vi "TemperatureDAQExample.vi"() -> ()   [LabVIEW 2024]
uses:
  <vilib>/Analysis/baseanly.llb/Mean (DBL).vi
  <vilib>/DAQmx/create/channels.llb/DAQmx Create Channel (AI-Temperature-Thermocouple).vi
  <vilib>/DAQmx/configure/trigger.llb/DAQmx Start Trigger (Digital Edge).vi
  <vilib>/Analysis/NI_AALBase.lvlib
  <vilib>/Utility/TDMS File Viewer/NI_TDMS File Viewer.lvlib
panel:
  out "data 4":dynamicdata(graph) caption="data"
  out "data 3":dynamicdata(graph) caption="data"
  out "mean":dbl format="%0.2f"
  in  "Boolean":bool
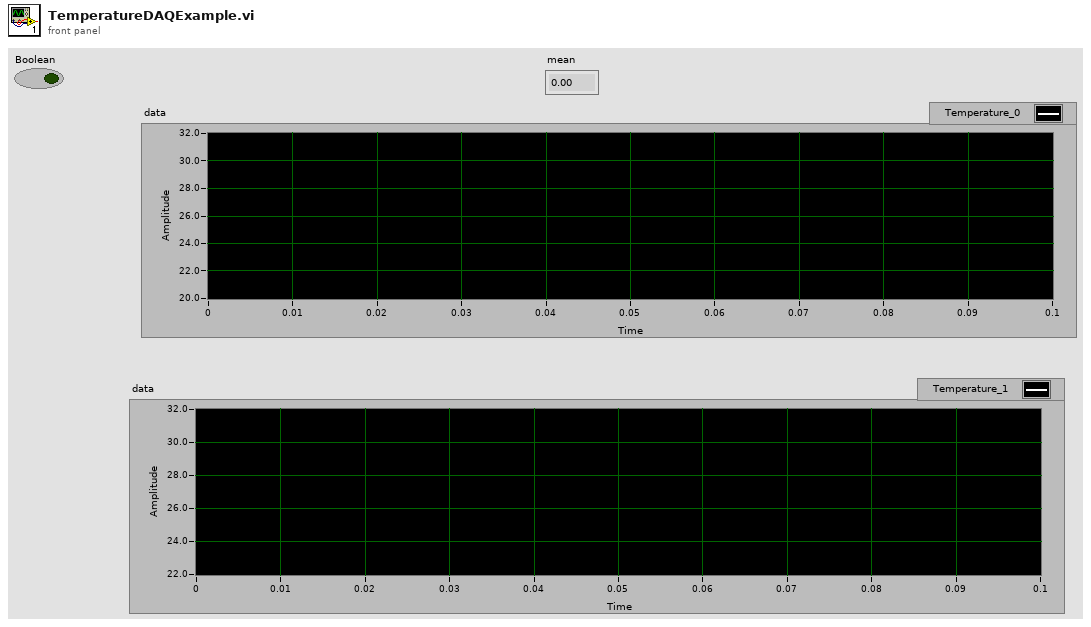
[diagram p1: front panel]
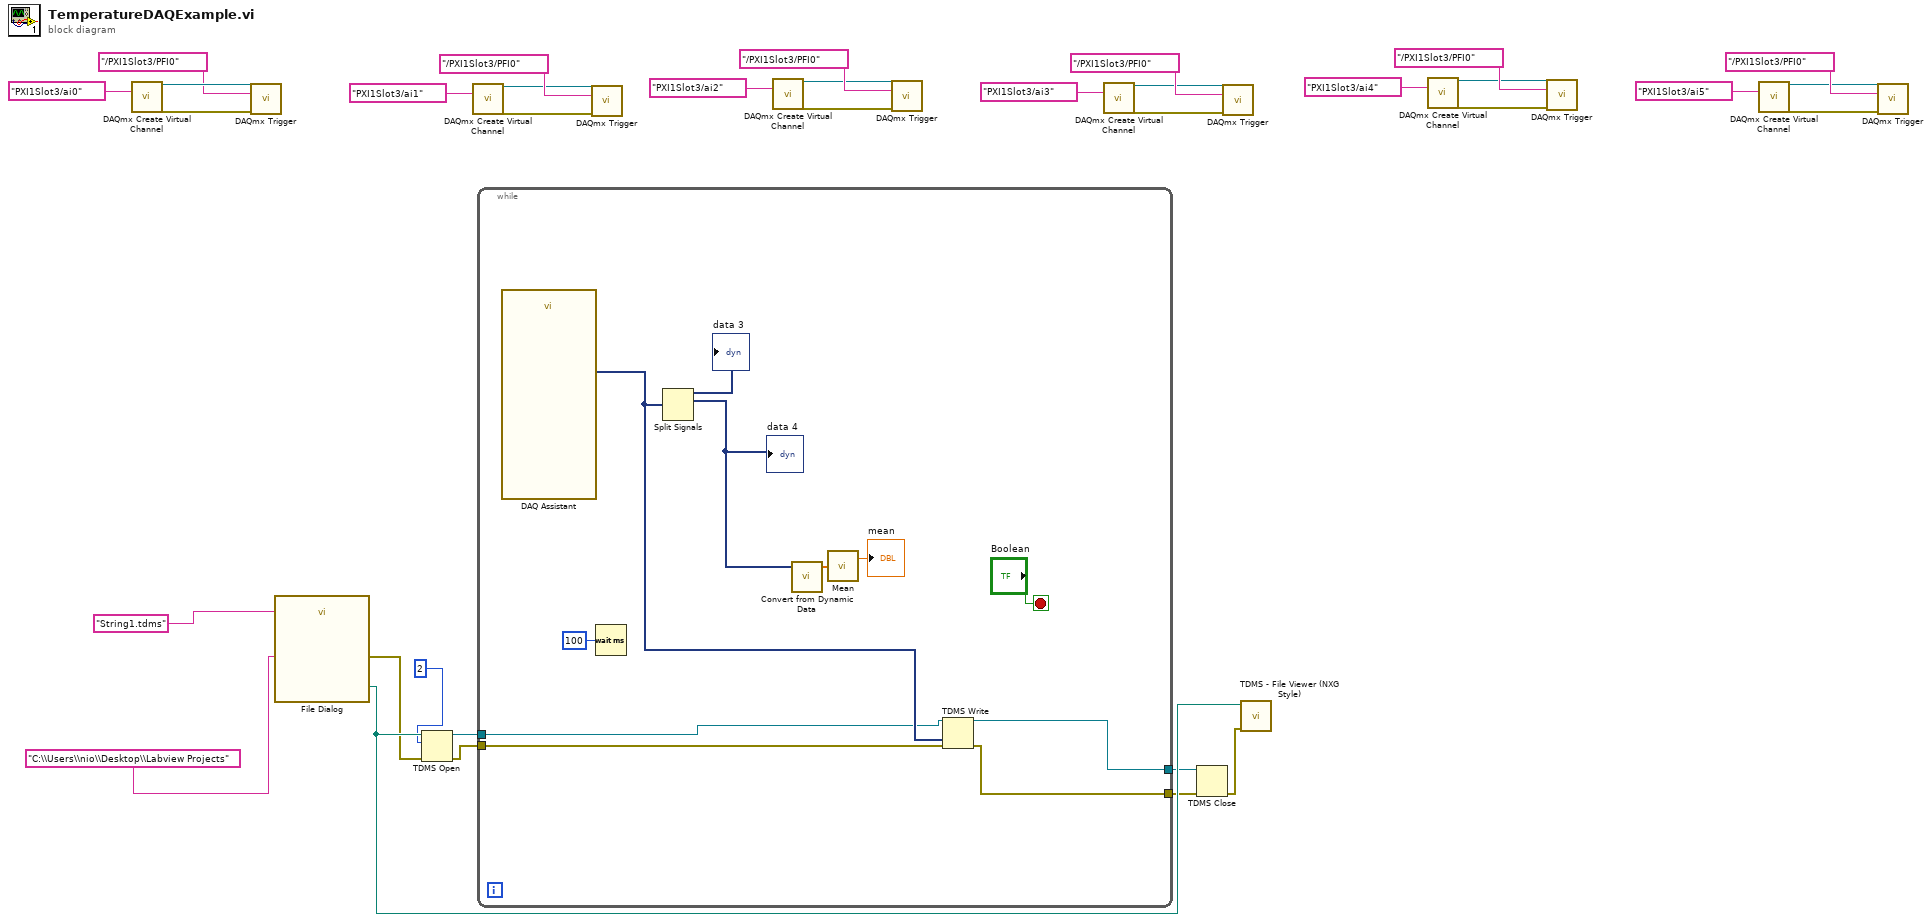
[diagram p0: block diagram]
diagram:
  n1 = call-poly <vilib>:"DAQmx Create Virtual Channel.vi"("physical channels"=tag "PXI1Slot3/ai0") -> ("task out"=w33:refnum<k21>, "error out"=w32:errorcluster)  [unwired: 13 in]
  n2 = call-poly <vilib>:"DAQmx Trigger.vi"("task/channels in"=w33, "source"=tag "/PXI1Slot3/PFI0", "error in"=w32) -> ()  [unwired: 11 in, 2 out]
  n3 = call "File Dialog"("prompt"="C:\\Users\\nio\\Desktop\\Labview Projects", "default name"="String1.tdms") -> ("selected path"=w24:path, "error out"=w23:errorcluster)  [unwired: 10 in, 2 out]
  n4 = TDMS Open(8:w23, 10:u32 2 ("milliseconds to wait"), 11:w24) -> (0:w21:errorcluster, 3:w20:refnum<k34>)  [unwired: 4 in]
  n5 = call-poly <vilib>:"DAQmx Create Virtual Channel.vi"("physical channels"=tag "PXI1Slot3/ai1") -> ("task out"=w27:refnum<k21>, "error out"=w29:errorcluster)  [unwired: 13 in]
  n6 = while {
    tunnel: w21 -> [w38]
    tunnel: w20 -> [w37]
    tunnel: [w36] -> w19
    tunnel: [w35] -> w18
    stop <- "Boolean" stop-if-true
    n7 = call "DAQ Assistant"() -> ("data"=w39:dynamicdata)  [unwired: 17 in, 2 out]
    n8 = Wait (ms)(milliseconds to wait=u32 100) -> ()  [unwired: 1 out]
    n9 = Split Signals(w39) -> (→"data 3":dynamicdata, w40:dynamicdata)  [unwired: 4 in, 2 out]
    "data 4" <- w40
    n10 = call "Convert from Dynamic Data"("Dynamic Data Type"=w40) -> ("Array"=w43:dbl[])  [unwired: 3 in]
    n11 = call-poly <vilib>:"Mean.vi"("X"=w43) -> ("mean"=→"mean":dbl)  [unwired: 1 out]
    n12 = TDMS Write(0:w37, 9:w39, 11:w38) -> (4:w35:refnum<k34>, 15:w36:errorcluster)  [unwired: 3 in, 2 out]
  }
  n13 = call-poly <vilib>:"DAQmx Trigger.vi"("task/channels in"=w27, "source"=tag "/PXI1Slot3/PFI0", "error in"=w29) -> ()  [unwired: 11 in, 2 out]
  n14 = call-poly <vilib>:"DAQmx Create Virtual Channel.vi"("physical channels"=tag "PXI1Slot3/ai2") -> ("task out"=w13:refnum<k21>, "error out"=w15:errorcluster)  [unwired: 13 in]
  n15 = call-poly <vilib>:"DAQmx Trigger.vi"("task/channels in"=w13, "source"=tag "/PXI1Slot3/PFI0", "error in"=w15) -> ()  [unwired: 11 in, 2 out]
  n16 = call-poly <vilib>:"DAQmx Create Virtual Channel.vi"("physical channels"=tag "PXI1Slot3/ai3") -> ("task out"=w9:refnum<k21>, "error out"=w11:errorcluster)  [unwired: 13 in]
  n17 = TDMS Close(8:w19, 11:w18) -> (0:w17:errorcluster)  [unwired: 1 out]
  n18 = call-poly <vilib>:"DAQmx Trigger.vi"("task/channels in"=w9, "source"=tag "/PXI1Slot3/PFI0", "error in"=w11) -> ()  [unwired: 11 in, 2 out]
  n19 = call <vilib>:"TDMS - File Viewer (NXG Style).vi"("error in"=w17, "file in"=w24) -> ()  [unwired: 8 in, 2 out]
  n20 = call-poly <vilib>:"DAQmx Create Virtual Channel.vi"("physical channels"=tag "PXI1Slot3/ai4") -> ("task out"=w5:refnum<k21>, "error out"=w7:errorcluster)  [unwired: 13 in]
  n21 = call-poly <vilib>:"DAQmx Trigger.vi"("task/channels in"=w5, "source"=tag "/PXI1Slot3/PFI0", "error in"=w7) -> ()  [unwired: 11 in, 2 out]
  n22 = call-poly <vilib>:"DAQmx Create Virtual Channel.vi"("physical channels"=tag "PXI1Slot3/ai5") -> ("task out"=w1:refnum<k21>, "error out"=w3:errorcluster)  [unwired: 13 in]
  n23 = call-poly <vilib>:"DAQmx Trigger.vi"("task/channels in"=w1, "source"=tag "/PXI1Slot3/PFI0", "error in"=w3) -> ()  [unwired: 11 in, 2 out]
